vi "Set Remote.vi"(0 "VISA Session In":refnum<visa-resource-name>="OXYMAT", 1 "Target Address":u8=16 format="%.0x", 2 "Source Address":u8=208 format="%.0x", 7 "Remote ON?":bool, 11 "error in (no error)":errorcluster) -> (4 "VISA Session Out":refnum<visa-resource-name>, 6 "Message Header":T1 {"Source Address" format="%.0x"; "Target Address" format="%.0x"}, 13 "Success":bool, 15 "error out":errorcluster)   [LabVIEW 2020, in "Siemens ELAN.lvlib"]
doc: "Using the Siemens ELAN protocol, sets the remote state ON or OFF (per the input boolean) on the addressed analyzer. Also returns a boolean indicating that the addressed device provided a valid response.\n\n$Revision:: 0 $\n$Modtime:: yy-mm-dd hh:mm $\n$Author:: Dboyd $"
uses:
  Siemens ELAN.lvlib
  Message Header.ctl
  Channel Status.ctl
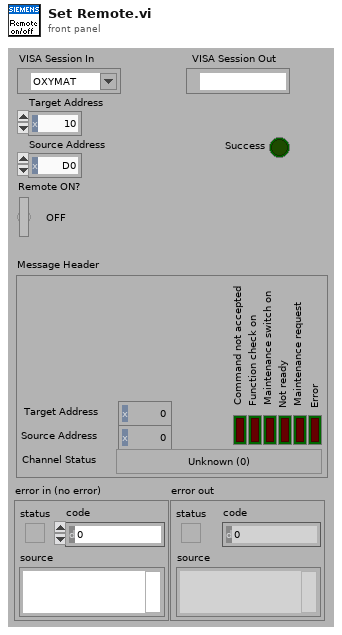
[diagram p1: front panel]
types:
  T1 = typedef "Siemens ELAN.lvlib/Message Header.ctl" = cluster{"Target Address":u8, "Source Address":u8, "Error":bool, "Maintenance request":bool, "Not ready":bool, "Maintenance switch on":bool, "Function check on":bool, "Command not accepted":bool, "Channel Status":T2}
  T2 = typedef "Siemens ELAN.lvlib/Channel Status.ctl" = enum8{"Unknown (0)", "Warm-up", "Pause", "Standby", "Measure", "Zero calibration", "Adjust component slope", "Unknown (7)", "Adjust curve dip", "Adjust linearization sensitivity", "Adjust temperature compensation", "Adjust pressure compensation", "Adjust linearization zero", "Adjust flow sensor", "Autocal", "Adjust phase", "Zero calibration of O2 sensor", "Synchronous zero calibration", "Purging for synchronous zero calibration", "Adjust analog output", "Adjust analog input", "Cleaning", "Unknown (>21)"}
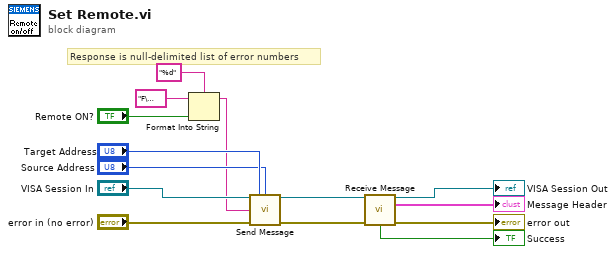
[diagram p0: block diagram]
diagram:
  # "Response is null-delimited list of error numbers"
  n1 = Format Into String(format string="%d", initial string="F\u0001" ("Command"), "Remote ON?") -> (resulting string=w1:string)  [unwired: 1 in, 1 out]
  n2 = call "Send Message.vi"("VISA Session In"="VISA Session In", "Target Address"="Target Address", "Source Address"="Source Address", "Command"=w1, "error in (no error)"="error in (no error)") -> ("VISA Session Out"=w14:refnum<visa-resource-name>, "error out"=w13:errorcluster)  [unwired: 8 in, 1 out]
  n3 = call "Receive Message.vi"("VISA Session In"=w14, "error in (no error)"=w13) -> ("VISA Session Out"=→"VISA Session Out":refnum<visa-resource-name>, "Message Header"=→"Message Header":T1, "Success"=→"Success":bool, "error out"=→"error out":errorcluster)  [unwired: 8 in, 2 out]
